vi "tempconfigXY.vi"(1 "Temp Config in":cluster{" XY":refnum<k21>, "E_XY":errorcluster}, 2 "command":string) -> (0 "Temp Config out":cluster{" XY":refnum<k21>, "E_XY":errorcluster})   [LabVIEW 2013]
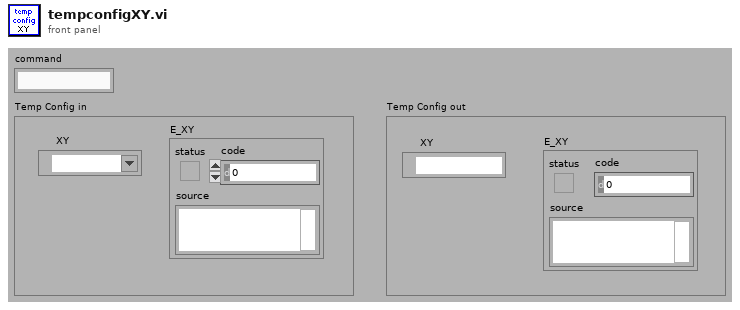
[diagram p1: front panel]
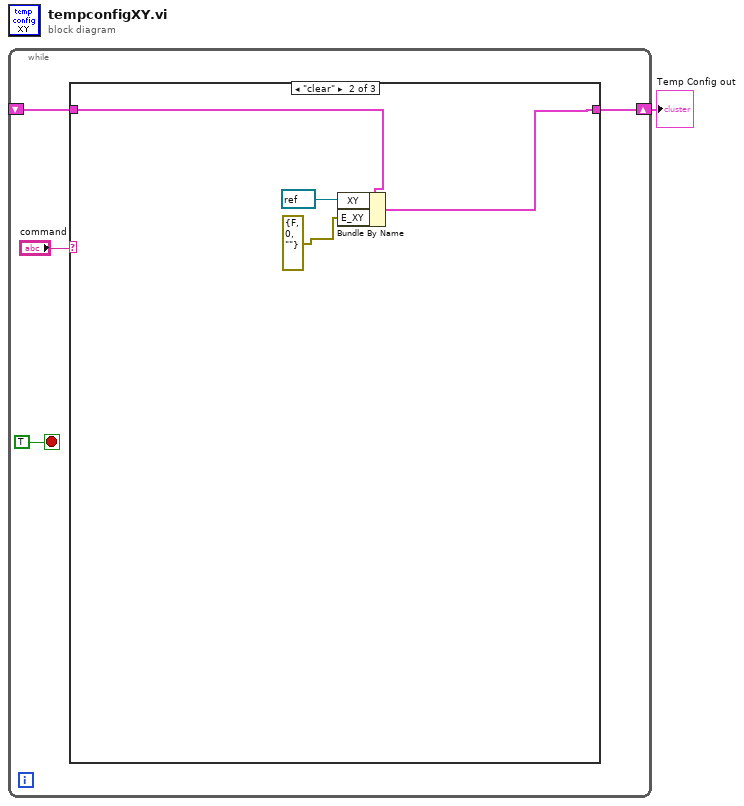
[diagram p0: block diagram]
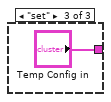
[diagram p3: hidden frame]
diagram:
  n1 = while {
    shift-right: [w3] -> w1
    shift-left: _ -> [w2]
    stop <- TRUE stop-if-true
    n2 = case shown="\"clear\"" "command" {
      tunnel: [w6 w9 "Temp Config in"] -> w3
      tunnel: w2 -> [w6 w10 _]
      frame "get", Default {
      }
      frame "clear" {
        n3 = Bundle By Name(cluster=w10, "XY"=refnum<k21> refnum, "E_XY"=errorcluster {"status"=FALSE, "code"=0, "source"=""} ("E_AI")) -> (w9:cluster{" XY":refnum<k21>, "E_XY":errorcluster})
      }
      frame "set" {
      }
    }
  }
  "Temp Config out" <- w1
